vi "Burning.vi"(0 "LT_UpgradeFlash in":refnum<class "LT_UpgradeFlash.lvclass">, 5 "burnFilePath":path=path "D:/Project/Tymphany/LT_UpgradeFlash/HDMI Board/LT FW  Files/LT9611 UXC/lt9611uxc_fw.bin", 7 "chipName":string, 9 "TimeOut(ms)":dbl, 11 "error in (no error)":errorcluster) -> (4 "LT_UpgradeFlash out":refnum<class "LT_UpgradeFlash.lvclass">, 6 "ActionResult":bool, 10 "resultStr":string, 15 "error out":errorcluster)   [LabVIEW 2017, in "LT_UpgradeFlash.lvclass"]
uses:
  LT_UpgradeFlash.lvclass
  D:/Project/Tymphany/LT_UpgradeFlash/LT_UpgradeFlash_dll/LT_UpgradeFlash_dll/bin/Debug/LT_UpgradeFlash_dll.dll
  LT_UpgradeFlash_dll/LT_UpgradeFlash_dll/bin/Debug/LT_UpgradeFlash_dll.dll
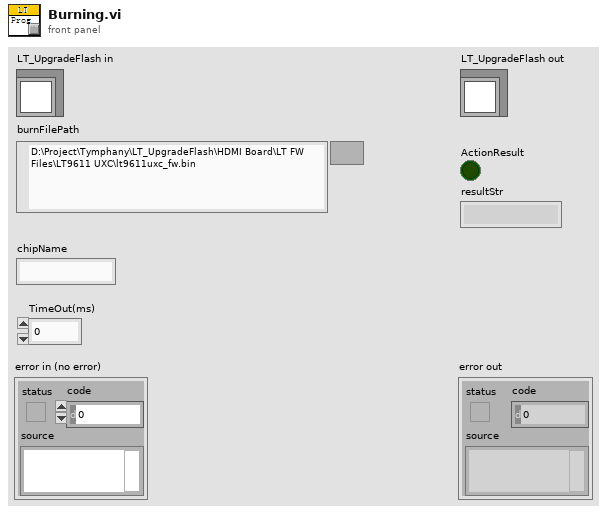
[diagram p1: front panel]
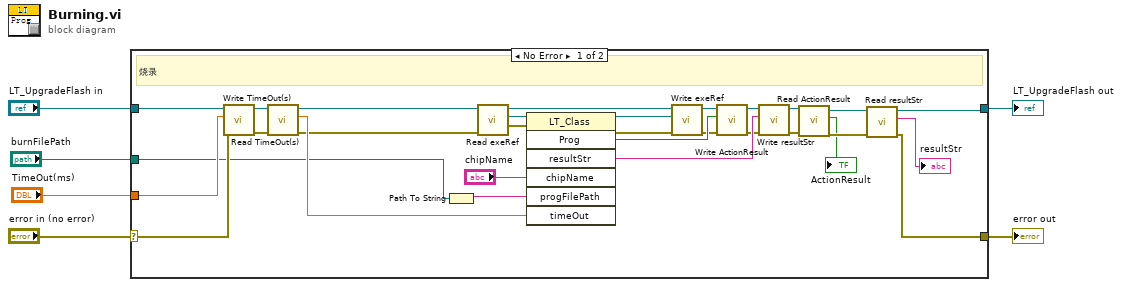
[diagram p0: block diagram]
diagram:
  n1 = case shown="No Error" "error in (no error)" {
    selector: "error in (no error)" -> [w24 w38]
    tunnel: [w16 w38] -> w5
    tunnel: [w17 w37] -> w3
    tunnel: "LT_UpgradeFlash in" -> [w25 w37]
    tunnel: "burnFilePath" -> [w7 _]
    tunnel: "TimeOut(ms)" -> [w13 _]
    frame No Error {
      # "烧录"
      n2 = call-dynamic "Write TimeOut(s).vi"("error in (no error)"=w24, "TimeOut(s)"=w13, "LT_UpgradeFlash in"=w25) -> ("error out"=w14:errorcluster, "LT_UpgradeFlash out"=w15:refnum<class "LT_UpgradeFlash.lvclass">)  [unwired: 7 in]
      n3 = call-dynamic "Read TimeOut(s).vi"("error in (no error)"=w14, "LT_UpgradeFlash in"=w15) -> ("error out"=w9:errorcluster, "TimeOut(s)"=w12:dbl, "LT_UpgradeFlash out"=w10:refnum<class "LT_UpgradeFlash.lvclass">)  [unwired: 7 in]
      n4 = Path To String(path=w7) -> (string=w11:string)
      n5 = call-dynamic "Read exeRef.vi"("error in (no error)"=w9, "LT_UpgradeFlash in"=w10) -> ("error out"=w32:errorcluster, "exeRef"=w36:refnum<k24>, "LT_UpgradeFlash out"=w26:refnum<class "LT_UpgradeFlash.lvclass">)  [unwired: 7 in]
      n6 = invoke class="LT_Class" method="Prog"(reference=w36, error in=w32, "chipName"="chipName", "progFilePath"=w11, "timeOut"=w12) -> (reference out=w35:refnum<k24>, error out=w31:errorcluster, "Prog"=w34:bool, "resultStr"=w33:string)  [unwired: 2 in, 3 out]
      n7 = call-dynamic "Write exeRef.vi"("error in (no error)"=w31, "exeRef"=w35, "LT_UpgradeFlash in"=w26) -> ("error out"=w29:errorcluster, "LT_UpgradeFlash out"=w30:refnum<class "LT_UpgradeFlash.lvclass">)  [unwired: 7 in]
      n8 = call-dynamic "Write ActionResult.vi"("error in (no error)"=w29, "ActionResult"=w34, "LT_UpgradeFlash in"=w30) -> ("error out"=w27:errorcluster, "LT_UpgradeFlash out"=w28:refnum<class "LT_UpgradeFlash.lvclass">)  [unwired: 7 in]
      n9 = call-dynamic "Write resultStr.vi"("error in (no error)"=w27, "resultStr"=w33, "LT_UpgradeFlash in"=w28) -> ("error out"=w18:errorcluster, "LT_UpgradeFlash out"=w19:refnum<class "LT_UpgradeFlash.lvclass">)  [unwired: 7 in]
      n10 = call-dynamic "Read ActionResult.vi"("error in (no error)"=w18, "LT_UpgradeFlash in"=w19) -> ("error out"=w22:errorcluster, "ActionResult"=→"ActionResult":bool, "LT_UpgradeFlash out"=w23:refnum<class "LT_UpgradeFlash.lvclass">)  [unwired: 7 in]
      n11 = call-dynamic "Read resultStr.vi"("error in (no error)"=w22, "LT_UpgradeFlash in"=w23) -> ("error out"=w16:errorcluster, "resultStr"=→"resultStr":string, "LT_UpgradeFlash out"=w17:refnum<class "LT_UpgradeFlash.lvclass">)  [unwired: 7 in]
    }
    frame Error {
    }
  }
  "error out" <- w5
  "LT_UpgradeFlash out" <- w3
